vi "uc480_ArrayToImage.vi"(8 "Error In":errorcluster, 10 "InArray":u8[](array[numeric]), 11 ".NET (Reference)":refnum<k24>) -> (0 "Error Out":errorcluster, 2 "Image":picture)   [LabVIEW 2011]
doc: "ArrayToVision converts 24/32-bit one-dimensional arrays to a two-dimensional U32 array."
uses:
  C:/Program Files/Thorlabs/Scientific Imaging/DCx Camera Support/Develop/DotNet/uc480DotNet.dll
  Develop/DotNet/uc480DotNet.dll
  <vilib>/picture/picture.llb/Draw True-Color Pixmap.vi
panel:
  # "Input"
  # "Output"
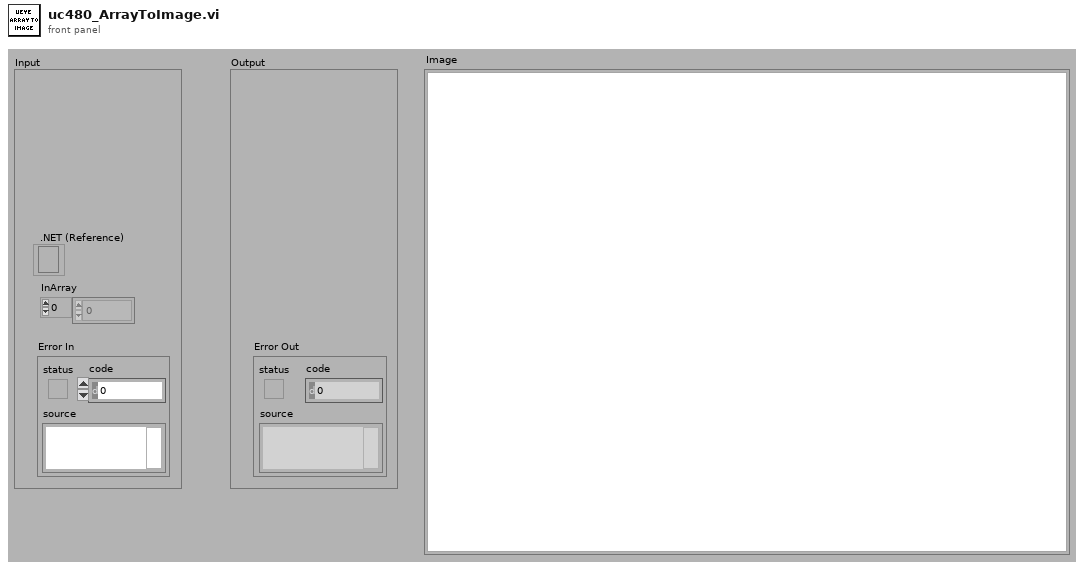
[diagram p1: front panel]
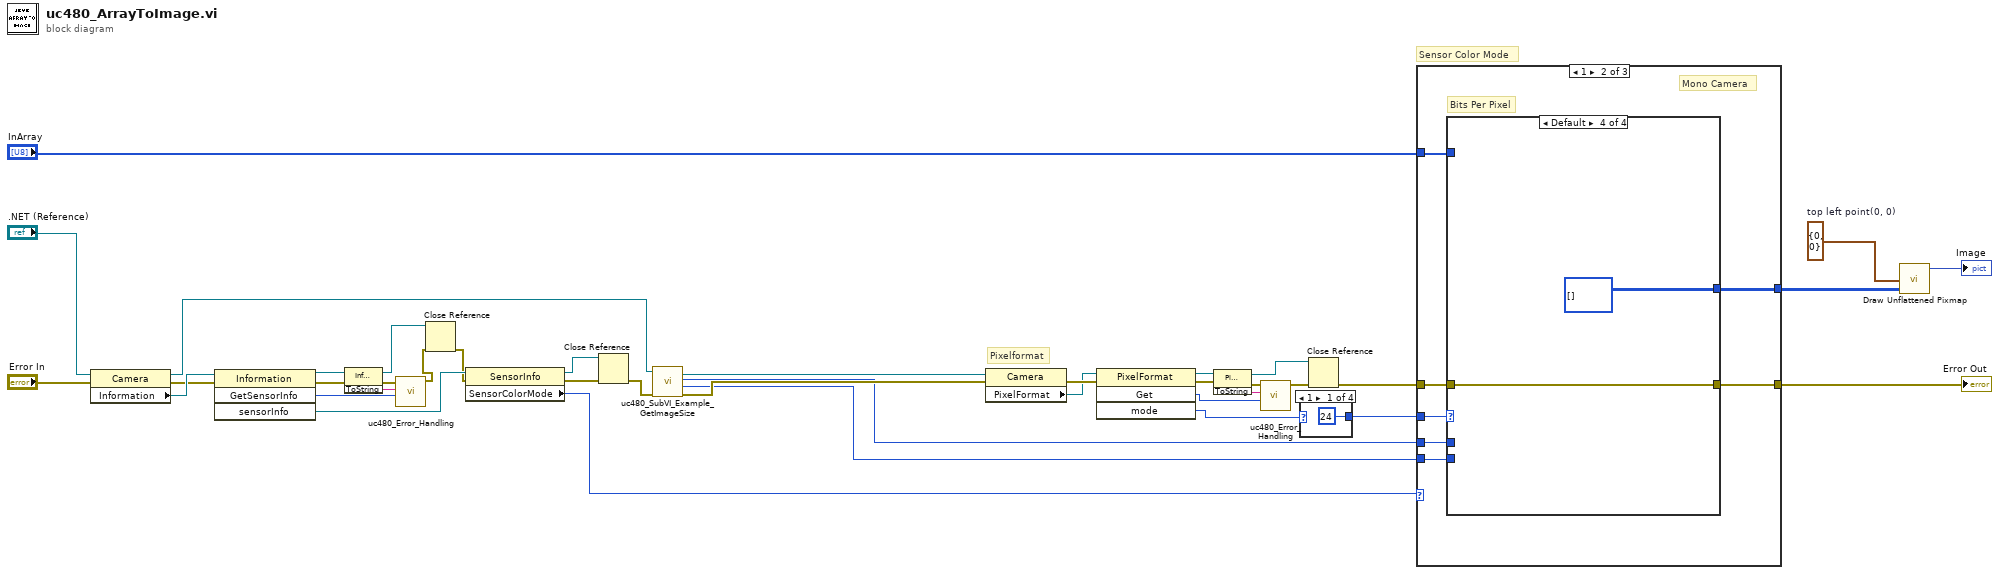
[diagram p0: block diagram]
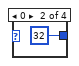
[diagram p2: hidden frame]
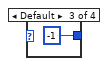
[diagram p3: hidden frame]
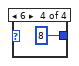
[diagram p4: hidden frame]
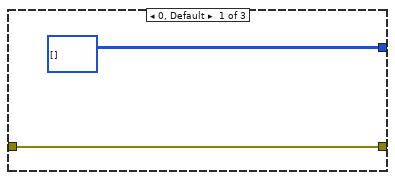
[diagram p5: hidden frame]
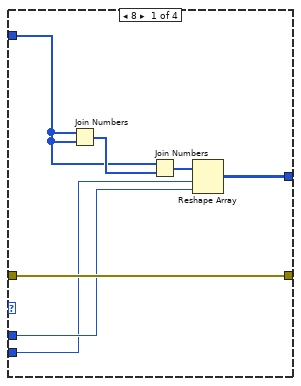
[diagram p6: hidden frame]
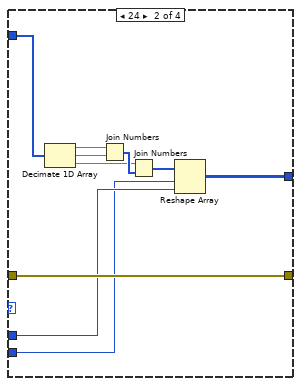
[diagram p7: hidden frame]
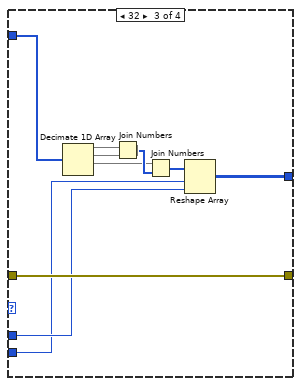
[diagram p8: hidden frame]
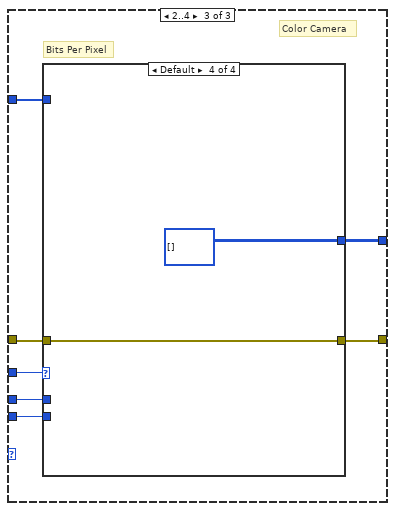
[diagram p9: hidden frame]
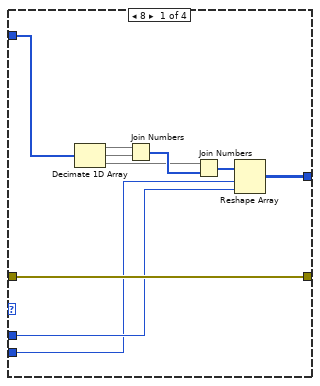
[diagram p10: hidden frame]
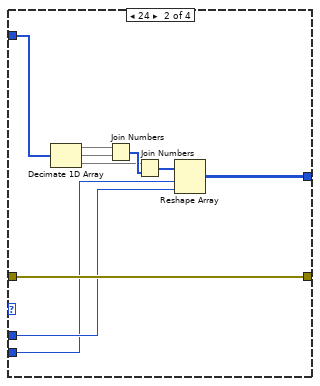
[diagram p11: hidden frame]
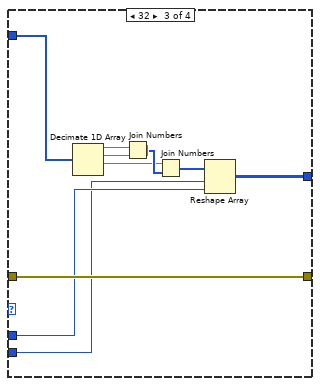
[diagram p12: hidden frame]
diagram:
  w39 = cluster{i16, i16} {0, 0}  # top left point(0, 0)
  # "Sensor Color Mode"
  # "Pixelformat"
  n1 = property on="Eigenschaftsknoten" class="Camera"(reference=".NET (Reference)", error in="Error In") -> (reference out=w1:refnum<k24>, error out=w34:errorcluster, "Information"=w37:refnum<k24>)
  n2 = invoke class="Information" method="GetSensorInfo"(reference=w37, error in=w34) -> (reference out=w29:refnum<k24>, error out=w28:errorcluster, "GetSensorInfo"=w27:i32, "sensorInfo"=w36:refnum<k24>)  [unwired: 2 in]
  n3 = invoke class="Information" method="ToString"(reference=w29, error in=w28) -> (reference out=w10:refnum<k24>, error out=w31:errorcluster, "ToString"=w30:string)  [unwired: 1 in]
  n4 = call "uc480_Error_Handling.vi"("Error Code"=w27, "Error String"=w30, "Error In"=w31) -> ("Error Out"=w9:errorcluster)  [unwired: 8 in]
  n5 = Close Reference(reference=w10, error in (no error)=w9) -> (error out=w8:errorcluster)
  n6 = property class="SensorInfo"(reference=w36, error in=w8) -> (reference out=w7:refnum<k24>, error out=w6:errorcluster, "SensorColorMode"=w35:i32)
  n7 = Close Reference(reference=w7, error in (no error)=w6) -> (error out=w5:errorcluster)
  n8 = call "uc480_SubVI_Example_GetImageSize.vi"("Error In"=w5, ".NET (Reference)"=w1) -> ("Error Out"=w15:errorcluster, "Height"=w11:i32, "Width"=w12:i32, ".NET (Reference)"=w13:refnum<k24>)  [unwired: 6 in]
  n9 = property class="Camera"(reference=w13, error in=w15) -> (error out=w21:errorcluster, "PixelFormat"=w20:refnum<k24>)  [unwired: 1 out]
  n10 = invoke class="PixelFormat" method="Get"(reference=w20, error in=w21) -> (reference out=w26:refnum<k24>, error out=w25:errorcluster, "Get"=w24:i32, "mode"=w19:i32)  [unwired: 2 in]
  n11 = invoke class="PixelFormat" method="ToString"(reference=w26, error in=w25) -> (reference out=w4:refnum<k24>, error out=w22:errorcluster, "ToString"=w23:string)  [unwired: 1 in]
  n12 = call "uc480_Error_Handling.vi"("Error Code"=w24, "Error String"=w23, "Error In"=w22) -> ("Error Out"=w3:errorcluster)  [unwired: 8 in]
  n13 = case shown="1" w19 {
    tunnel: [24 32 -1 8] -> w18
    frame 1 {
    }
    frame 0 {
    }
    frame Default {
    }
    frame 6 {
    }
  }
  n14 = Close Reference(reference=w4, error in (no error)=w3) -> (error out=w2:errorcluster)
  n15 = case shown="1" w35 {
    tunnel: "InArray" -> [_ w49 w88]
    tunnel: w12 -> [_ w47 w83]
    tunnel: w11 -> [_ w46 w82]
    tunnel: w18 -> [_ w48 w84]
    tunnel: w2 -> [w44 w52 w85]
    tunnel: [w44 w51 w86] -> w17
    tunnel: [u32[][] [] w50 w87] -> w16
    frame 0, Default {
    }
    frame 1 {
      # "Bits Per Pixel"
      # "Mono Camera"
      n16 = case shown="Default" w48 {
        tunnel: w49 -> [w55 w64 w73 _]
        tunnel: w46 -> [w53 w60 w70 _]
        tunnel: w47 -> [w54 w61 w71 _]
        tunnel: [w59 w63 w74 u32[][] []] -> w50
        tunnel: w52 -> [w58 w62 w72 w80]
        tunnel: [w58 w62 w72 w80] -> w51
        frame 8 {
          n17 = Join Numbers(hi=w55, lo=w55) -> ((hi.lo)=w57:u16[])
          n18 = Join Numbers(hi=w55, lo=w57) -> ((hi.lo)=w56:u32[])
          n19 = Reshape Array(w56, w53, w54) -> (w59:u32[][])
        }
        frame 24 {
          n20 = Decimate 1D Array(w64) -> (w69:u8[], w68:u8[], w66:u8[])
          n21 = Join Numbers(hi=w68, lo=w69) -> ((hi.lo)=w67:u16[])
          n22 = Join Numbers(hi=w66, lo=w67) -> ((hi.lo)=w65:u32[])
          n23 = Reshape Array(w65, w60, w61) -> (w63:u32[][])
        }
        frame 32 {
          n24 = Decimate 1D Array(w73) -> (w79:u8[], w78:u8[], w76:u8[])  [unwired: 1 out]
          n25 = Join Numbers(hi=w78, lo=w79) -> ((hi.lo)=w77:u16[])
          n26 = Join Numbers(hi=w76, lo=w77) -> ((hi.lo)=w75:u32[])
          n27 = Reshape Array(w75, w70, w71) -> (w74:u32[][])
        }
        frame Default {
        }
      }
    }
    frame 2..4 {
      # "Bits Per Pixel"
      # "Color Camera"
      n28 = case shown="Default" w84 {
        tunnel: w88 -> [w90 w103 w112 _]
        tunnel: w82 -> [w95 w99 w109 _]
        tunnel: w83 -> [w96 w100 w110 _]
        tunnel: [w98 w102 w113 u32[][] []] -> w87
        tunnel: w85 -> [w97 w101 w111 w119]
        tunnel: [w97 w101 w111 w119] -> w86
        frame 8 {
          n29 = Decimate 1D Array(w90) -> (w94:u8[], w93:u8[], w91:u8[])
          n30 = Join Numbers(hi=w93, lo=w94) -> ((hi.lo)=w92:u16[])
          n31 = Join Numbers(hi=w91, lo=w92) -> ((hi.lo)=w89:u32[])
          n32 = Reshape Array(w89, w95, w96) -> (w98:u32[][])
        }
        frame 24 {
          n33 = Decimate 1D Array(w103) -> (w108:u8[], w107:u8[], w105:u8[])
          n34 = Join Numbers(hi=w107, lo=w108) -> ((hi.lo)=w106:u16[])
          n35 = Join Numbers(hi=w105, lo=w106) -> ((hi.lo)=w104:u32[])
          n36 = Reshape Array(w104, w99, w100) -> (w102:u32[][])
        }
        frame 32 {
          n37 = Decimate 1D Array(w112) -> (w118:u8[], w117:u8[], w115:u8[])  [unwired: 1 out]
          n38 = Join Numbers(hi=w117, lo=w118) -> ((hi.lo)=w116:u16[])
          n39 = Join Numbers(hi=w115, lo=w116) -> ((hi.lo)=w114:u32[])
          n40 = Reshape Array(w114, w109, w110) -> (w113:u32[][])
        }
        frame Default {
        }
      }
    }
  }
  "Error Out" <- w17
  n41 = call-poly <vilib>:"Draw Unflattened Pixmap.vi"("top left point(0, 0)"=w39, "data (RGB format)"=w16) -> ("new picture"=→"Image":picture)  [unwired: 7 in]
